vi "test objective.vi"(9 "output selector":T1, 10 "data":variant, 11 "X":dbl[](array[numeric])) -> (0 "error out":errorcluster, 1 "inequality constraint function values":dbl[](array[numeric]), 2 "equality constraint function values":dbl[](array[numeric]), 3 "objective function value":dbl)   [LabVIEW 2020]
doc: "This template is the starting point for creating an objective function, equality constraint function and inequality constraint function to be passed to the Constrained Nonlinear Optimization.vi."
uses:
  <vilib>/gmath/NumericalOptimization/cno_output select.ctl
  <vilib>/gmath/NI_Gmath.lvlib
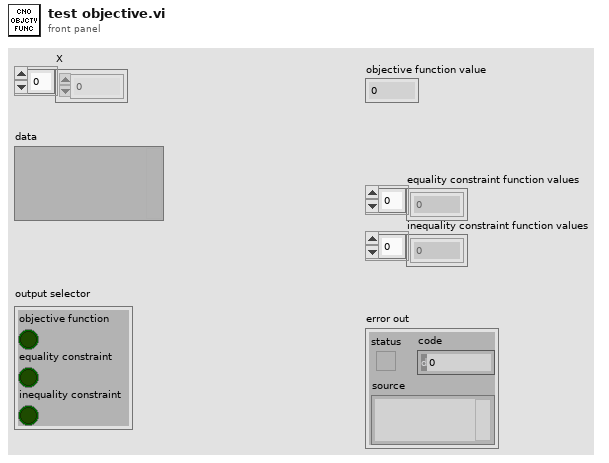
[diagram p1: front panel]
types:
  T1 = typedef "NI_Gmath.lvlib/cno_output select.ctl" = cluster{"objective function":bool, "equality constraint":bool, "inequality constraint":bool}
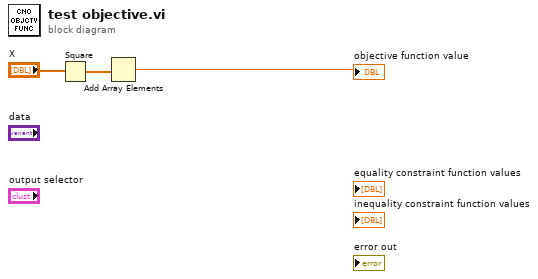
[diagram p0: block diagram]
diagram:
  n1 = Square(x="X") -> (x^2=w2:dbl[])
  n2 = Add Array Elements(numeric array=w2) -> (sum=→"objective function value":dbl)
